vi "FG_Message_Queue.vi"(7 "Action":T1, 8 "error in":errorcluster) -> (0 "error out":errorcluster, 3 "Message Queue":refnum<queue>)   [LabVIEW 2014]
uses:
  Typedef_Message_Queue_Action.ctl
  support/Message Queue/Message Cluster.ctl
  support/Message Queue/Message Queue.lvlib
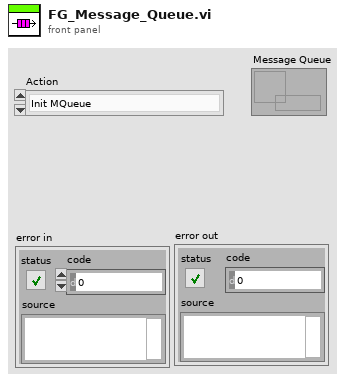
[diagram p1: front panel]
types:
  T1 = typedef "Typedef_Message_Queue_Action.ctl" = enum16{"Init MQueue", "Get MQueue Ref", "Close MQueue"}
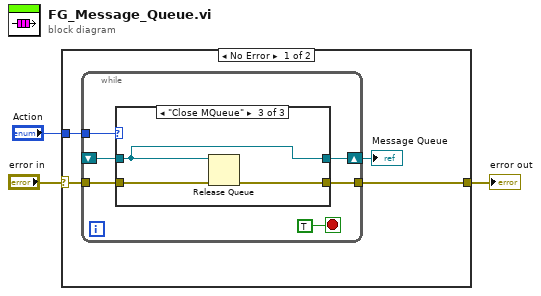
[diagram p0: block diagram]
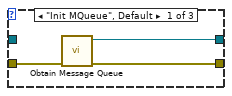
[diagram p2: hidden frame]
diagram:
  n1 = case shown="No Error" "error in" {
    selector: "error in" -> [w7 w22]
    tunnel: [w5 w22] -> w2
    tunnel: "Action" -> [w6 _]
    frame No Error {
      n2 = while {
        tunnel: w7 -> [w11]
        tunnel: w6 -> [w12]
        shift-right: [w9] -> w4
        shift-left: _ -> [w10]
        tunnel: [w8] -> w5
        stop <- TRUE stop-if-true
        n3 = case shown="\"Close MQueue\"" w12 {
          tunnel: w11 -> [w16 w17 w21]
          tunnel: w10 -> [_ w18 w19]
          tunnel: [w15 w18 w19] -> w9
          tunnel: [w14 w17 w20] -> w8
          frame "Init MQueue", Default {
            n4 = call "Obtain Message Queue.vi"("error in (no error)"=w16) -> ("error out"=w14:errorcluster, "Message Queue"=w15:refnum<queue>)  [unwired: 9 in]
          }
          frame "Get MQueue Ref" {
          }
          frame "Close MQueue" {
            n5 = Release Queue(queue=w19, error in (no error)=w21) -> (error out=w20:errorcluster)  [unwired: 1 in, 2 out]
          }
        }
      }
      "Message Queue" <- w4
    }
    frame Error {
    }
  }
  "error out" <- w2
